vi "Read Module Menu Name.vi"(8 "error in":errorcluster, 11 "UI Reference editor node in":refnum<class "UI Reference editor node.lvclass">) -> (0 "error out":errorcluster, 2 "Menu Name":string, 3 "UI Reference editor node out":refnum<class "UI Reference editor node.lvclass">)   [LabVIEW 2013, in "UI Reference editor node.lvclass"]
uses:
  UI Reference editor node.lvclass
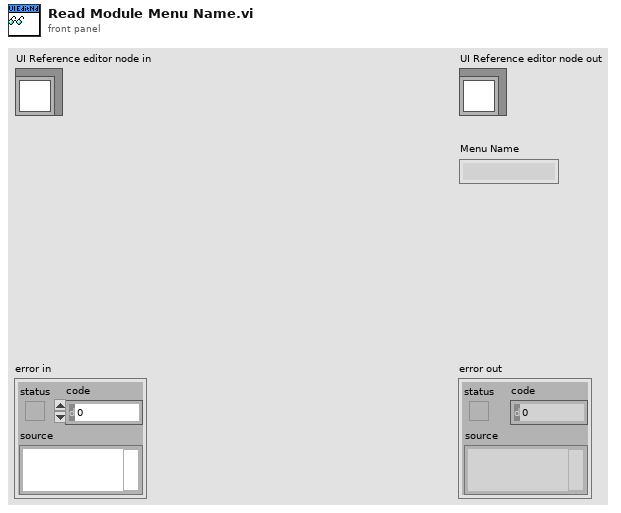
[diagram p1: front panel]
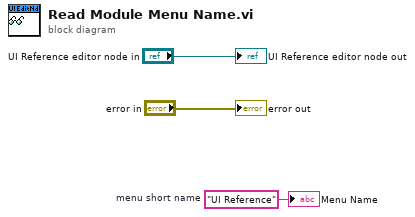
[diagram p0: block diagram]
diagram:
  w1 = "UI Reference"  # menu short name
  "error out" <- "error in"
  "UI Reference editor node out" <- "UI Reference editor node in"
  "Menu Name" <- w1
